vi "Final.vi"() -> ()   [LabVIEW 2025]
uses:
  <vilib>/Instr/_visa.llb/VISA Configure Serial Port (Instr).vi
  <vilib>/Utility/file.llb/Read Delimited Spreadsheet (string).vi
  <vilib>/httpClient/POSTBuffer.vi
  <vilib>/httpClient/LabVIEWHTTPClient.lvlib
panel:
  in  "stop":bool
  in  "VISA resource name":refnum<visa-resource-name>
  out "Grafic Inregistrare Persoane":waveform(i16)[](graph)
  out "Output":T1(array[cluster]) {"Timp inregistrat (s)" format="%#_2g"}
  out "Waveform":waveform(i32)
  out "element":T2
  in  "Cluster 2":T2
  out "current time 2":timestamp
  in  "Active timers":T3(array[cluster])
  in  "Last Elapsed":dbl
  in  "Cluster":T2
  in  "UID":string[](array[string])
  in  "Array":string[](array[string])
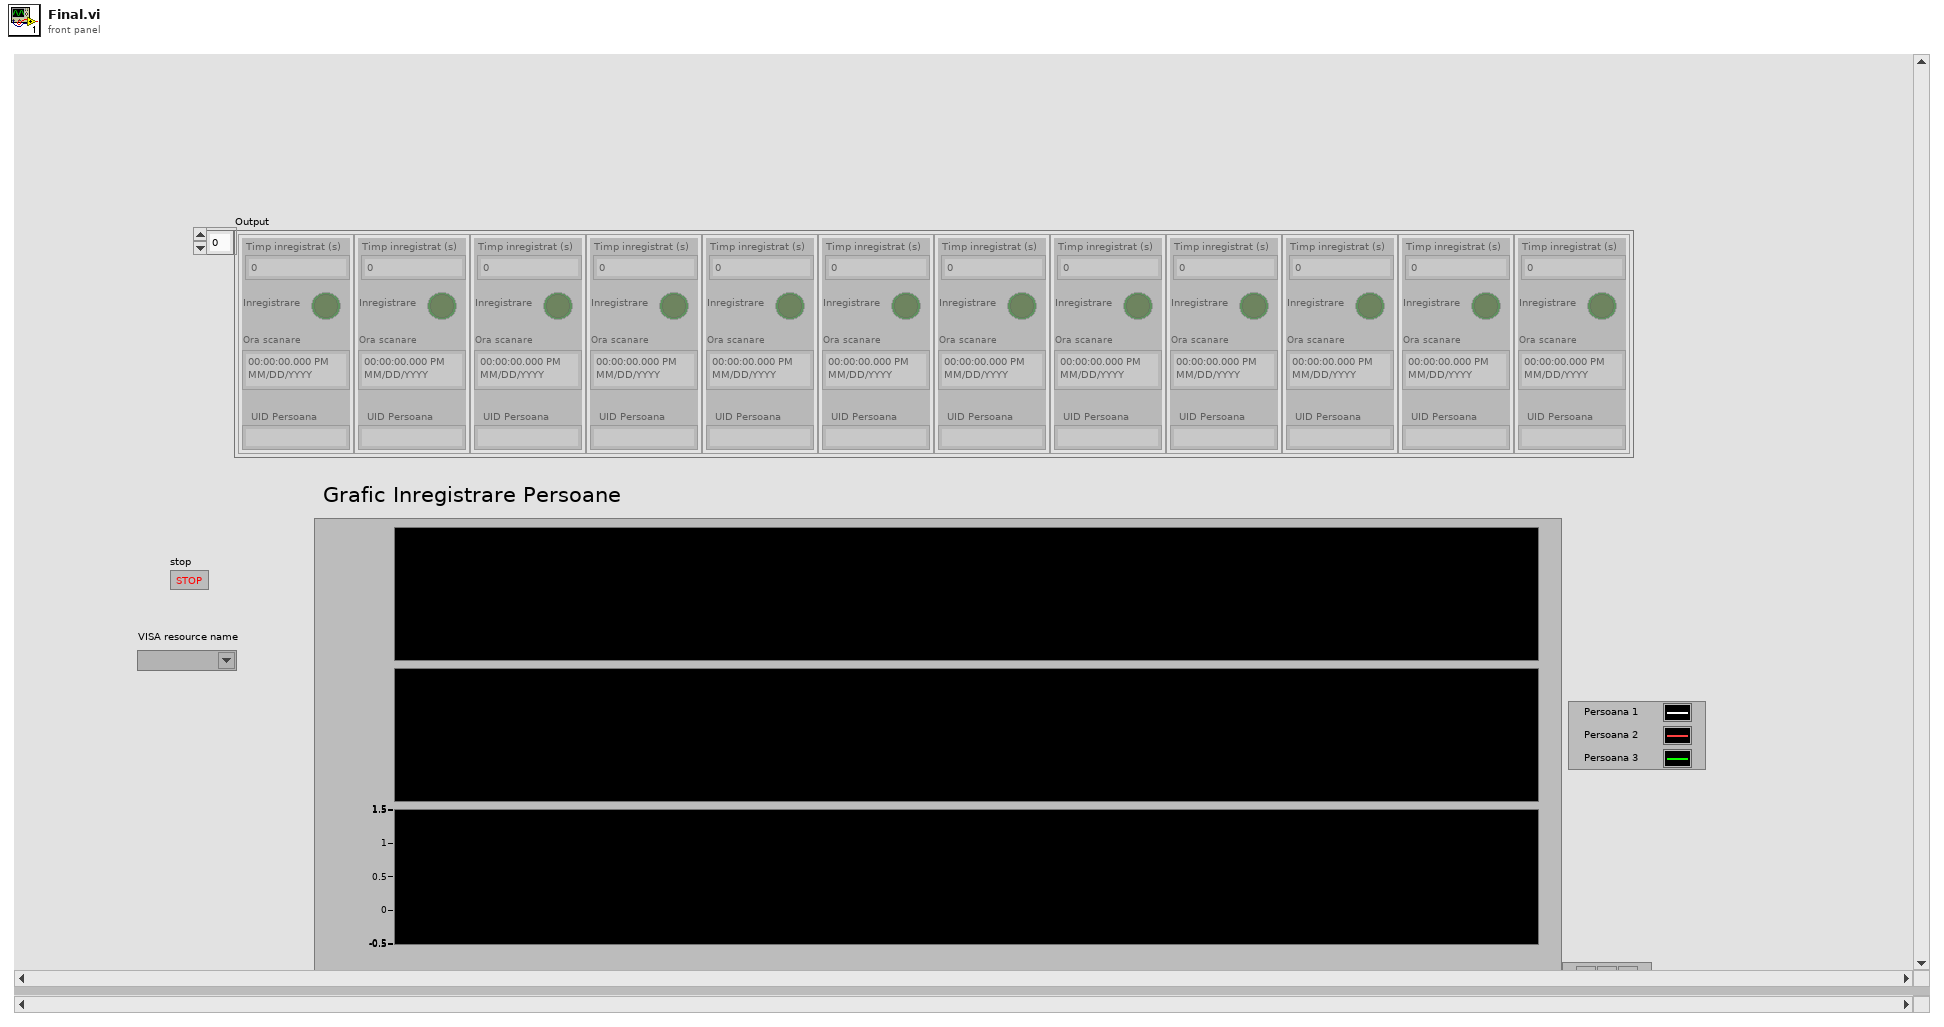
[diagram p1: front panel]
types:
  T1 = cluster{"Timp inregistrat (s)":dbl, "Inregistrare":bool, "Ora scanare":timestamp, "UID Persoana":string}[]
  T2 = cluster{"Last Elapsed":dbl, "Running":bool, "current time":timestamp, "String":string}
  T3 = cluster{"Last Elapsed":dbl, "Running":bool, "current time":timestamp, "String":string}[]
  T4 = enum16{"open", "replace", "create", "open or create", "replace or create", "replace or create with confirmation"}
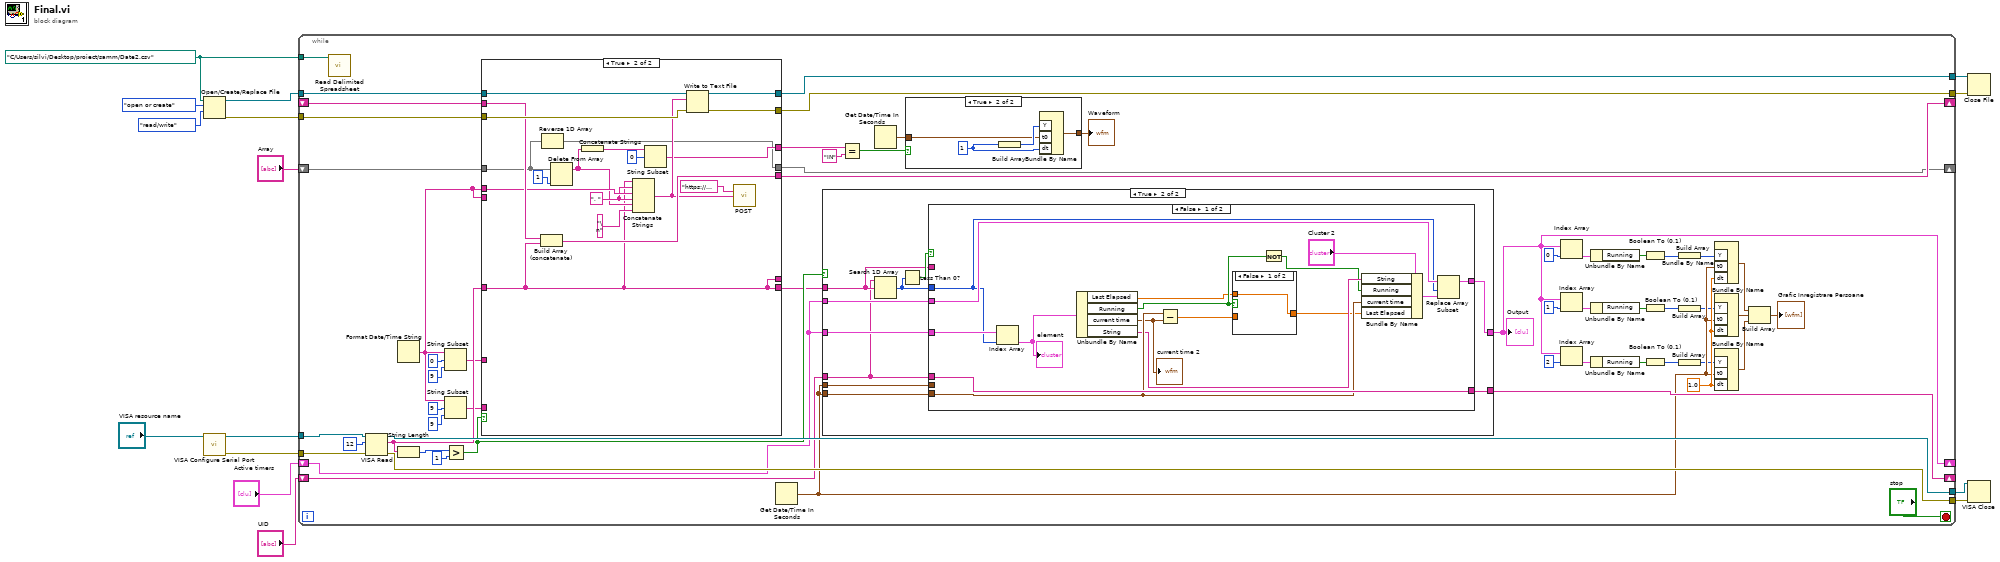
[diagram p0: block diagram]
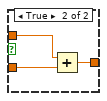
[diagram p3: hidden frame]
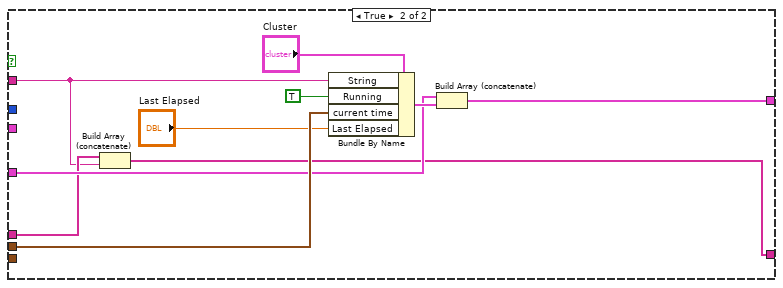
[diagram p4: hidden frame]
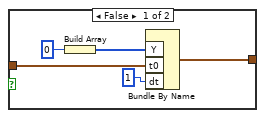
[diagram p5: hidden frame]
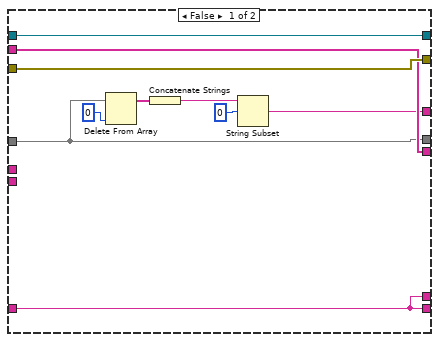
[diagram p6: hidden frame]
diagram:
  w4 = path "C:/Users/silvi/Desktop/proiect/samm/Date2.csv" ("file path (use dialog)")
  n1 = Open/Create/Replace File(file path (use dialog)=w4, operation (0:open)=T4."open or create", access (0:read/write)=enum16{"read/write", "read-only", "write-only"}."read/write") -> (refnum out=w8:refnum<file>, error out=w7:errorcluster)  [unwired: 3 in, 1 out]
  n2 = call-poly "VISA Configure Serial Port"("VISA resource name"="VISA resource name") -> ("VISA resource name out"=w11:refnum<visa-resource-name>, "error out"=w14:errorcluster)  [unwired: 13 in]
  n3 = while {
    tunnel: w14 -> [w72]
    tunnel: [w71] -> w13
    tunnel: [w70] -> w12
    tunnel: w11 -> [w68]
    shift-right: [w65] -> _
    shift-left: _ -> [w64]
    tunnel: w8 -> [w62]
    tunnel: w7 -> [w61]
    tunnel: [w60] -> w6
    tunnel: [w59] -> w5
    tunnel: w4 -> [w46]
    shift-right: [w47] -> _
    shift-left: "Array" -> [w48]
    shift-right: [w37] -> _
    shift-left: "UID" -> [w42]
    shift-right: [w35] -> _
    shift-left: "Active timers" -> [w41]
    stop <- "stop" stop-if-true
    w25 = 1.0 ("dt")
    n4 = call-poly <vilib>:"Read Delimited Spreadsheet.vi"("file path (dialog if empty)"=w46) -> ()  [unwired: 9 in, 6 out]
    n5 = VISA Read(VISA resource name=w68, byte count=u32 12, error in (no error)=w72) -> (VISA resource name out=w71:refnum<visa-resource-name>, read buffer=w63:string, error out=w70:errorcluster)  [unwired: 1 out]
    n6 = Format Date/Time String() -> (date/time string=w52:string)  [unwired: 3 in]
    n7 = String Length(string=w63) -> (length=w67:i32)
    n8 = String Subset(string=w52, offset (0)=0, length (rest)=9 ("length (rest)")) -> (substring=w53:string)
    n9 = String Subset(string=w52, offset (0)=9, length (rest)=9 ("length (rest)")) -> (substring=w54:string)
    n10 = Greater?(x=w67, y=1) -> (0:w44:bool)
    n11 = case shown="True" w44 {
      tunnel: w64 -> [w131 w148]
      tunnel: w63 -> [w124 w134]
      tunnel: [w131 w145] -> w65
      tunnel: w62 -> [w133 w152]
      tunnel: w61 -> [w132 w151]
      tunnel: [w133 w150] -> w60
      tunnel: [w132 w149] -> w59
      tunnel: w52 -> [_ _]
      tunnel: w53 -> [_ _]
      tunnel: w54 -> [_ _]
      tunnel: w52 -> [_ w146]
      tunnel: [w124 w134] -> _
      tunnel: [w126 w140] -> w49
      tunnel: w48 -> [w128 w138]
      tunnel: [w128 w139] -> w47
      tunnel: [w124 w134] -> w43
      frame False {
        n12 = Delete From Array(array=w128, index=0) -> (array with subset deleted=w127:string[])  [unwired: 1 in, 1 out]
        n13 = Concatenate Strings(w127) -> (w129:string)
        n14 = String Subset(string=w129, offset (0)=0) -> (substring=w126:string)  [unwired: 1 in]
      }
      frame True {
        w144 = ", " ("string")
        n15 = Build Array (concatenate)(w148, w134) -> (w145:string[])
        n16 = Reverse 1D Array(array=w138) -> (reversed array=w139:string[])
        n17 = Delete From Array(array=w138, index=1) -> (array with subset deleted=w136:string[])  [unwired: 1 in, 1 out]
        n18 = Concatenate Strings(w136) -> (w135:string)
        n19 = Concatenate Strings(w134, w144, w146, w144, w136, "\n" ("string")) -> (w142:string)
        n20 = String Subset(string=w135, offset (0)=0) -> (substring=w140:string)  [unwired: 1 in]
        n21 = Write to Text File(file (use dialog)=w152, text=w142, error in=w151) -> (refnum out=w150:refnum<file>, error out=w149:errorcluster)  [unwired: 1 in, 1 out]
        n22 = call-poly <vilib>:"POST.vi"("url"="https://script.google.com/macros/s/AKfycbzDbFU9D64yF_qV9BctQEgvhDYqeG-a8-QBr04IH16IfWFLakNcDkjQtBWt9nd38Lif/exec", "buffer"=w142) -> ()  [unwired: 10 in, 4 out]
      }
    }
    n23 = Get Date/Time In Seconds() -> (seconds since 1Jan1904=w21:timestamp)
    n24 = case shown="True" w44 {
      tunnel: w42 -> [w73 w76]
      tunnel: w43 -> [_ w83]
      tunnel: w41 -> [w74 w82]
      tunnel: w21 -> [_ w81]
      tunnel: w21 -> [_ w79]
      tunnel: w41 -> [_ w78]
      tunnel: [w74 w77] -> w35
      tunnel: [w73 w75] -> w37
      frame False {
      }
      frame True {
        n25 = Search 1D Array(1D array=w76, element=w83) -> (index of element=w80:i32)  [unwired: 1 in]
        n26 = Less Than 0?(x=w80) -> (x < 0?=w84:bool)
        n27 = case shown="False" w84 {
          tunnel: w83 -> [_ w105]
          tunnel: w82 -> [w100 w111]
          tunnel: w81 -> [_ w114]
          tunnel: w80 -> [w90 _]
          tunnel: w79 -> [w94 _]
          tunnel: w78 -> [w97 _]
          tunnel: [w96 w110] -> w77
          tunnel: w76 -> [w95 w106]
          tunnel: [w95 w109] -> w75
          frame False {
            n28 = Index Array(array=w100, index=w90) -> (element=w99:T2)
            "element" <- w99
            n29 = Unbundle By Name(w99) -> ("Last Elapsed"=w87:dbl, "Running"=w89:bool, "current time"=w93:timestamp, "String"=w91:string)
            "current time 2" <- w93
            n30 = Subtract(x=w94, y=w93) -> (x-y=w88:dbl)
            n31 = case shown="False" w89 {
              tunnel: w88 -> [_ w104]
              tunnel: w87 -> [w101 w103]
              tunnel: [w101 w102] -> w86
              frame False {
              }
              frame True {
                n32 = Add(x=w103, y=w104) -> (x+y=w102:dbl)
              }
            }
            n33 = Not(x=w89) -> (.not. x?=w85:bool)
            n34 = Bundle By Name(cluster="Cluster 2", "String"=w91, "Running"=w85, "current time"=w94, "Last Elapsed"=w86) -> (w98:T2)
            n35 = Replace Array Subset(array=w97, new element=w98, index=w90) -> (w96:T3)
          }
          frame True {
            n36 = Build Array (concatenate)(w106, w105) -> (w109:string[])
            n37 = Bundle By Name(cluster="Cluster", "String"=w105, "Running"=TRUE, "current time"=w114, "Last Elapsed"="Last Elapsed") -> (w112:T2)
            n38 = Build Array (concatenate)(w111, w112) -> (w110:T3)
          }
        }
      }
    }
    "Output" <- w35
    n39 = Equal?(x=w49, y="IN") -> (x = y?=w50:bool)
    n40 = Get Date/Time In Seconds() -> (seconds since 1Jan1904=w45:timestamp)
    n41 = case shown="True" w50 {
      tunnel: [w116 w121] -> w16
      tunnel: w45 -> [w115 w120]
      frame False {
        n42 = Build Array(0 ("length (rest)")) -> (w119:i32[])
        n43 = Bundle By Name("Y"=w119, "t0"=w115, "dt"=1 ("length (rest)")) -> (w116:waveform(i32))  [unwired: 1 in]
      }
      frame True {
        w122 = 1 ("length (rest)")
        n44 = Build Array(w122) -> (w123:i32[])
        n45 = Bundle By Name("Y"=w123, "t0"=w120, "dt"=w122) -> (w121:waveform(i32))  [unwired: 1 in]
      }
    }
    "Waveform" <- w16
    n46 = Index Array(array=w35, index=0) -> (element=w39:T2)
    n47 = Index Array(array=w35, index=1) -> (element=w32:T2)
    n48 = Index Array(array=w35, index=2) -> (element=w33:T2)
    n49 = Unbundle By Name(w39) -> ("Running"=w38:bool)
    n50 = Unbundle By Name(w32) -> ("Running"=w31:bool)
    n51 = Unbundle By Name(w33) -> ("Running"=w30:bool)
    n52 = Boolean To (0,1)(Boolean=w38) -> (0, 1=w27:i16)
    n53 = Boolean To (0,1)(Boolean=w31) -> (0, 1=w28:i16)
    n54 = Boolean To (0,1)(Boolean=w30) -> (0, 1=w29:i16)
    n55 = Build Array(w27) -> (w19:i16[])
    n56 = Build Array(w28) -> (w18:i16[])
    n57 = Build Array(w29) -> (w17:i16[])
    n58 = Bundle By Name("Y"=w19, "t0"=w21, "dt"=w25) -> (w24:waveform(i16))  [unwired: 1 in]
    n59 = Bundle By Name("Y"=w18, "t0"=w21, "dt"=w25) -> (w23:waveform(i16))  [unwired: 1 in]
    n60 = Bundle By Name("Y"=w17, "t0"=w21, "dt"=w25) -> (w22:waveform(i16))  [unwired: 1 in]
    n61 = Build Array(w24, w23, w22) -> (→"Grafic Inregistrare Persoane":waveform(i16)[])
  }
  n62 = Close File(refnum=w6, error in=w5) -> ()  [unwired: 2 out]
  n63 = VISA Close(VISA resource name=w13, error in (no error)=w12) -> ()  [unwired: 1 out]
